vi "Facade.vi"(0 "Data In":T6={"t0"=timestamp(0 s since 1904-01-01), "dt"=0.0, "Y"=[]}, 2 "Display State In":T4, 3 "Container State":T5) -> (6 "Data Out":T6, 7 "Display State Out":T4, 8 "Action":T3)   [LabVIEW 2018, in "Waveform Control.xctl"]
uses:
  Waveform Control.xctl
  Controls/Data.ctl
  <vilib>/_xctls/Container State.ctl
  Controls/State.ctl
  <vilib>/_xctls/Action.ctl
  subvis/FP Controls.ctl
  subvis/Function Types.ctl
  Controls/Volatile State Ops.ctl
  <vilib>/_xctls/XControlSupport.lvlib
panel:
  in  "Controls":T1={"Type"=enum."Sine", "Periods"=0.0, "Points"=2, "Offset"=0.0, "Amplitdue"=0.0, "Starting Phase"=0.0, "func"=""} {"Points" min=1 step=1}
  out "Display":waveform(dbl)[](graph)
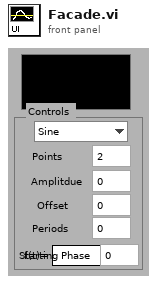
[diagram p1: front panel]
types:
  T1 = typedef "Waveform Control.xctl/FP Controls.ctl" = cluster{"Type":T2, "Periods":dbl, "Points":i32, "Offset":dbl, "Amplitdue":dbl, "Starting Phase":dbl, "func":string}
  T2 = typedef "Waveform Control.xctl/Function Types.ctl" = enum16{"Level", "Sine", "Triangle", "Ramp", "Saw Tooth", "Square", "Function"}
  T3 = typedef "XControlSupport.lvlib/Action.ctl" = cluster{"Data Changed?":bool, "State Changed?":bool, "Action Name":string}
  T4 = typedef "Waveform Control.xctl/State.ctl" = cluster{"Name":string}
  T5 = typedef "XControlSupport.lvlib/Container State.ctl" = cluster{"Indicator?":bool, "Run Mode?":bool, " Refnum":refnum<vi>}
  T6 = typedef "Waveform Control.xctl/Data.ctl" = waveform(dbl)
  T7 = typedef "Waveform Control.xctl/Volatile State Ops.ctl" = enum16{"Read", "Write", "Update State from Data"}
  T8 = typedef "Waveform Control.xctl/Waveform State.ctl" = cluster{"Show Axes":bool, "Show Y=0":bool, "Controls":T1, "Show Current Location":bool, "Current Location":i32, "dt":dbl, "t0":timestamp, "Amplitude Format String":string}
  T9 = typedef "LVRectTypeDef.ctl" = cluster{"Left":i16, "Top":i16, "Right":i16, "Bottom":i16}
  T10 = cluster{"Starting Phase":refnum<vi>, "Amplitdue":refnum<vi>, "Points":refnum<vi>, "Type":refnum<vi>, "Periods":refnum<vi>, "func":refnum<vi>, "Offset":refnum<vi>}
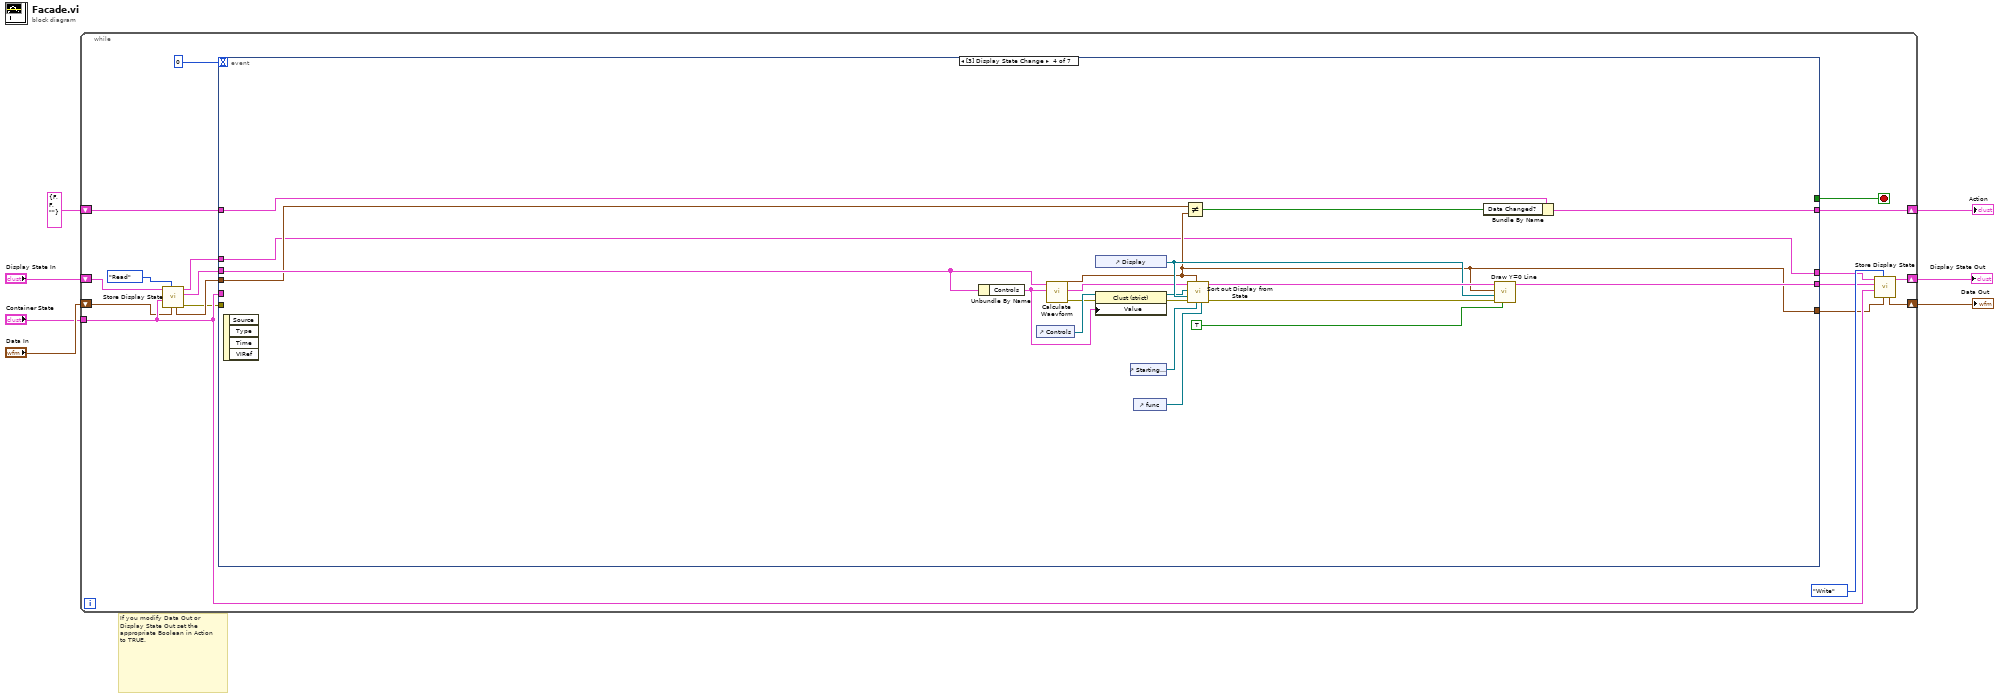
[diagram p0: block diagram]
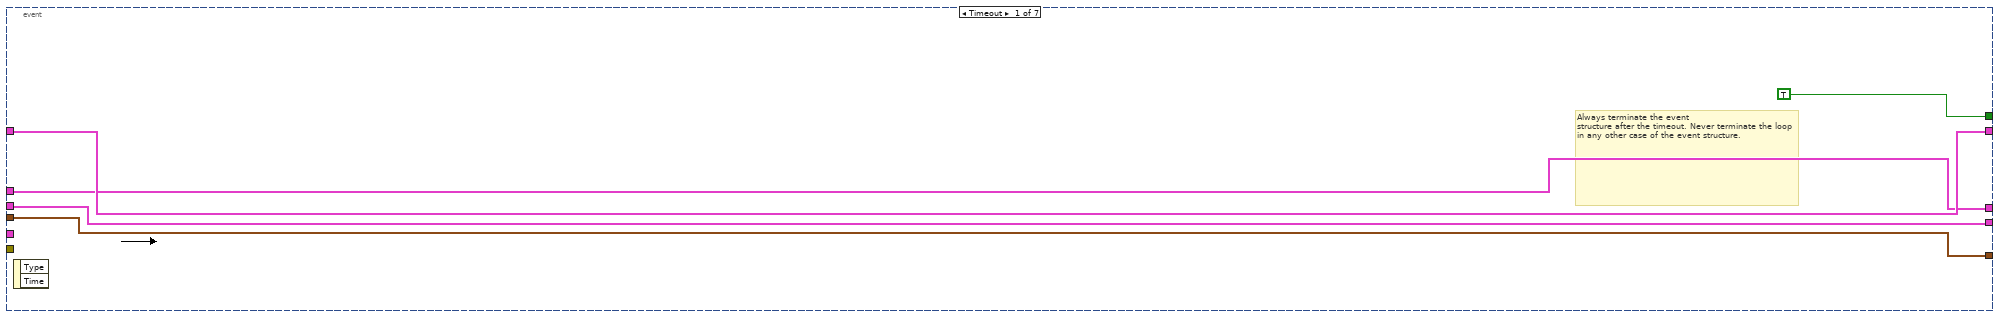
[diagram p2: hidden frame]
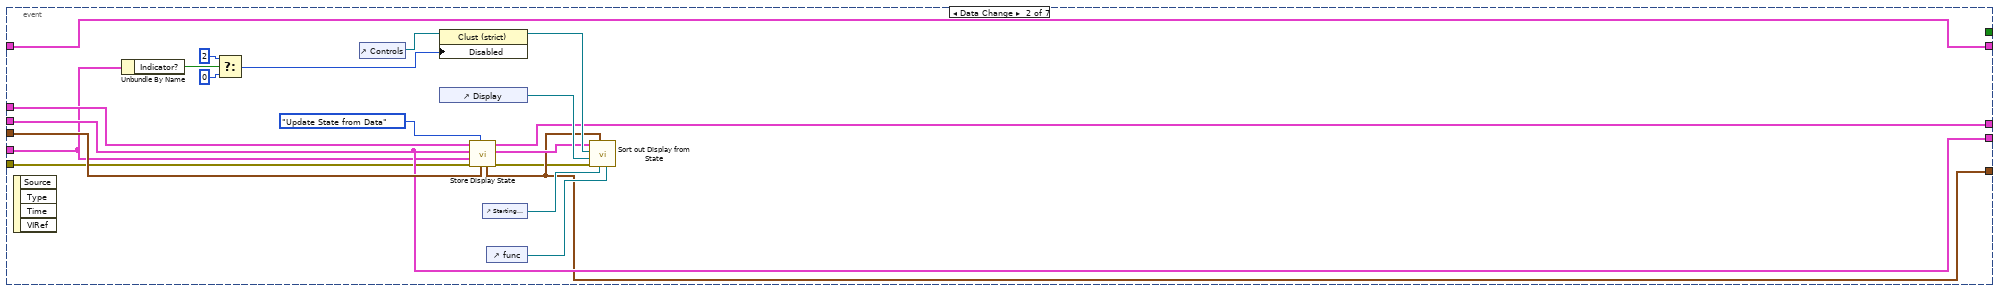
[diagram p3: hidden frame]
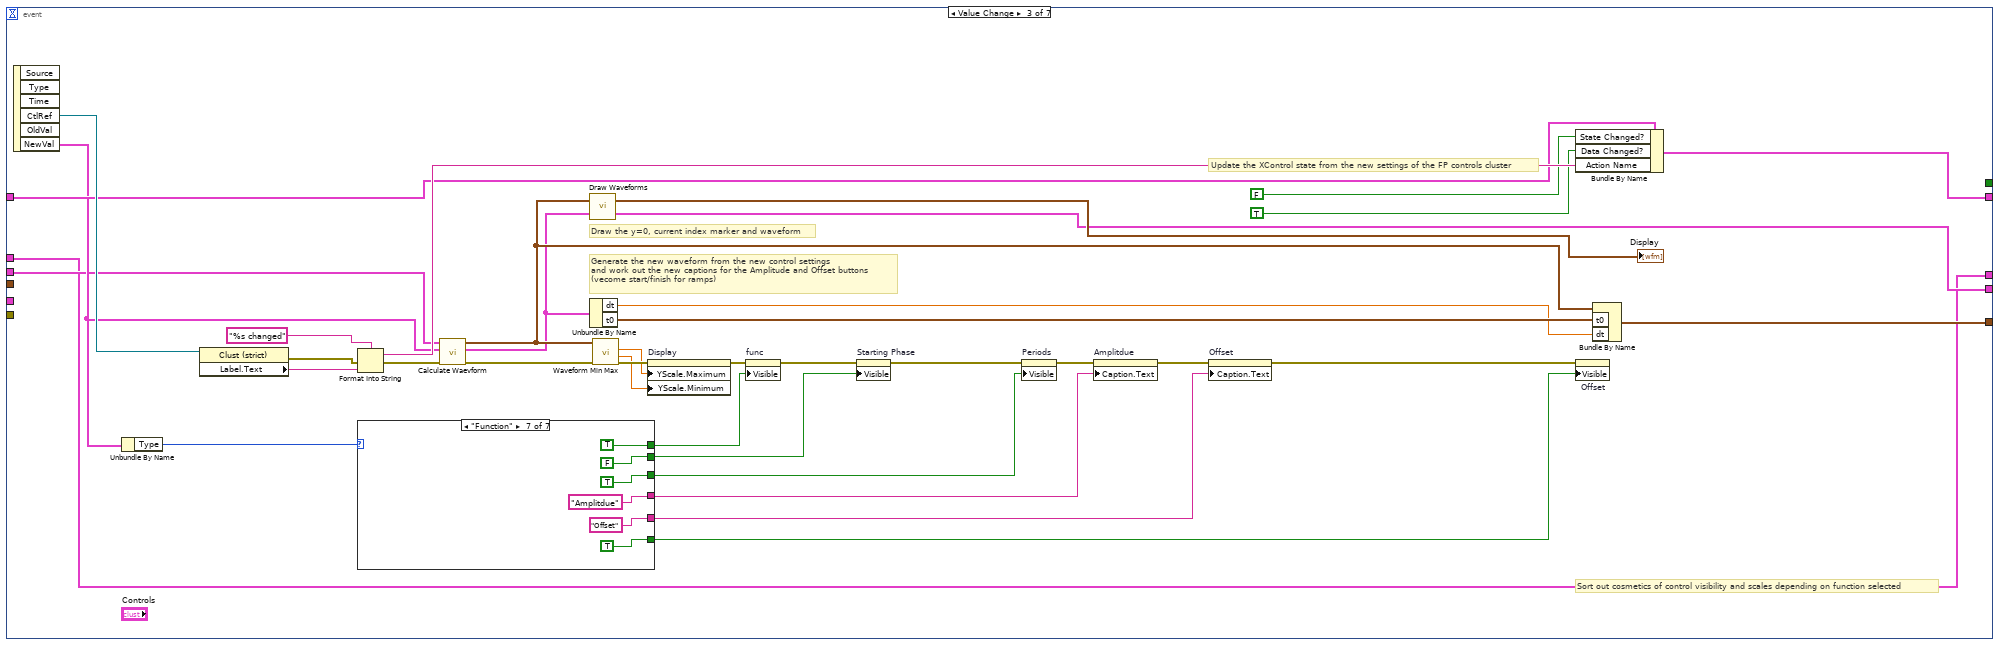
[diagram p4: hidden frame]
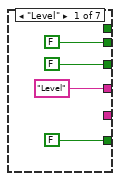
[diagram p5: hidden frame]
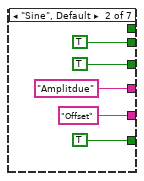
[diagram p6: hidden frame]
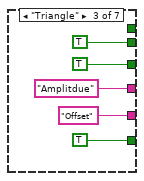
[diagram p7: hidden frame]
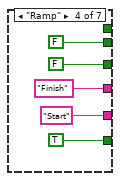
[diagram p8: hidden frame]
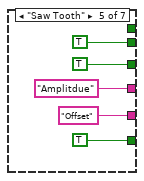
[diagram p9: hidden frame]
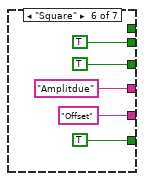
[diagram p10: hidden frame]
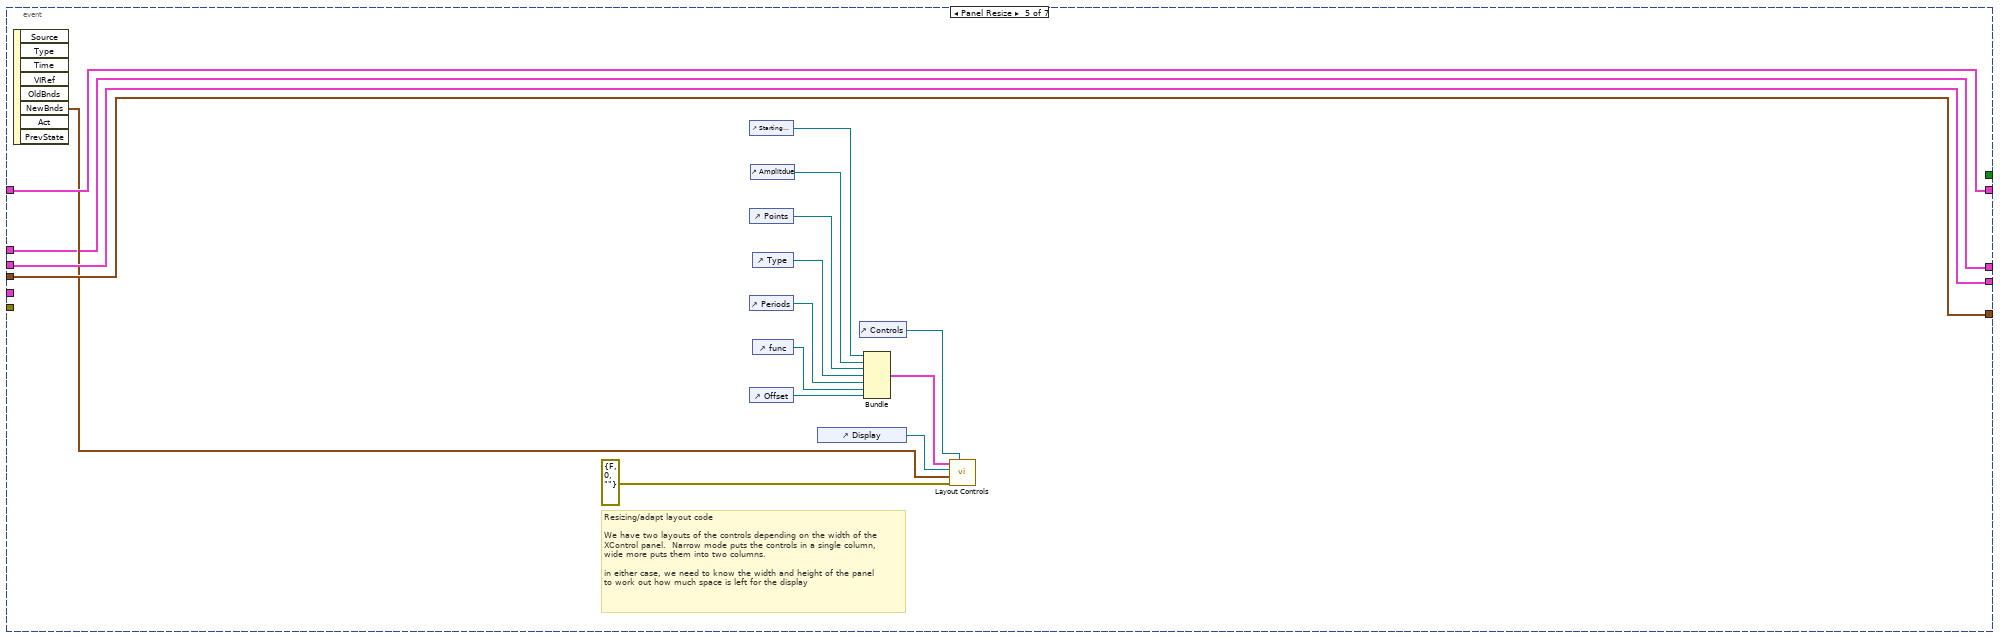
[diagram p11: hidden frame]
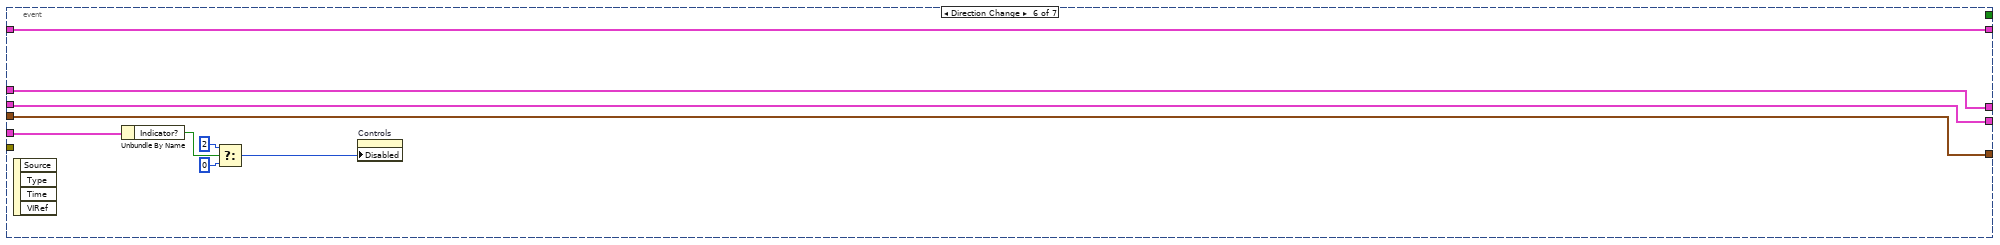
[diagram p12: hidden frame]
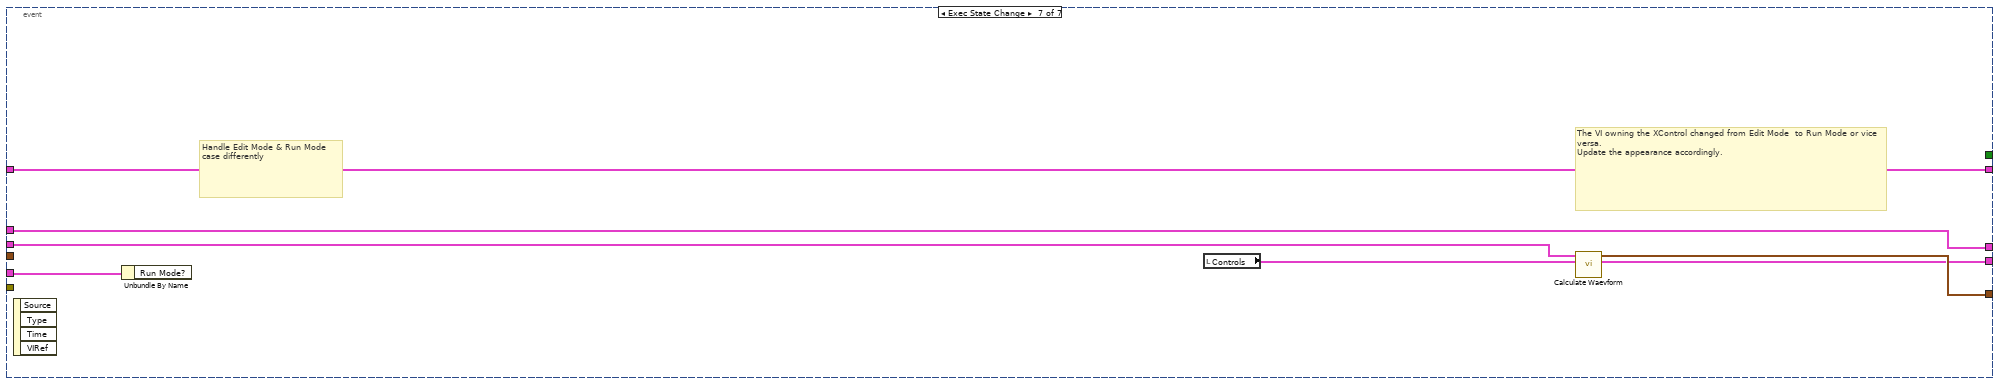
[diagram p13: hidden frame]
diagram:
  # "If you modify Data Out or\nDisplay State Out set the\nappropriate Boolean in Action\nto TRUE."
  n1 = while {
    shift-right: [w20] -> w4
    shift-left: "Display State In" -> [w25]
    tunnel: "Container State" -> [w15]
    shift-right: [w11] -> w7
    shift-left: "Data In" -> [w14]
    shift-right: [w21] -> w2
    shift-left: T3 {"Data Changed?"=FALSE, "State Changed?"=FALSE, "Action Name"=""} ("Action") -> [w22]
    stop <- w24 stop-if-true
    n2 = call "Store Display State.vi"("Data"=w14, "Operation In"=Volatile_State_Ops."Read", "Container State In"=w15, "State In"=w25) -> ("Error Out"=w8:errorcluster, "Waveform State Out"=w18:T8, "Display State Out"=w10:T4, "Data 2"=w13:T6)  [unwired: 2 in, 2 out]
    n3 = event shown="[3] Display State Change" {
      selector: _ -> [_ _ _ _ _ _ _]
      dyn-events: _ -> [_ _ _ _ _ _ _]
      timeout: 0 -> [_ _ _ _ _ _ _]
      tunnel: w18 -> [w28 w38 w54 w133 w157 w166 w169]
      tunnel: [w28 w38 w55 w134 w157 w166 w170] -> w17
      tunnel: [TRUE _ _ _ _ _ _] -> w24
      tunnel: w15 -> [_ w31 _ _ _ w167 w174]
      tunnel: w13 -> [w27 w40 _ w127 w158 w165 _]
      tunnel: [w27 w36 w62 w128 w158 w165 w171] -> w12
      tunnel: [w29 w32 w66 w141 w156 w164 w173] -> w21
      tunnel: w22 -> [w29 w32 w67 w142 w156 w164 w173]
      tunnel: w10 -> [w26 w41 w51 w125 w143 w159 w168]
      tunnel: [w26 w39 w51 w125 w143 w159 w168] -> w9
      tunnel: w8 -> [_ w33 _ _ _ _ _]
      event Timeout {
        # "Always terminate the event\nstructure after the timeout. Never terminate the loop in any other case of the event structure."
        n4 = event-data() -> ()  [unwired: 3 out]
      }
      event Data Change {
        n5 = event-data() -> ()  [unwired: 5 out]
        n6 = Unbundle By Name(w31) -> ("Indicator?"=w43:bool)
        n7 = Select(t=2, s=w43, f=0) -> (s? t:f=w46:i32)
        n8 = control-ref of="Controls"() -> (w50:refnum<vi>)
        n9 = property class="Clust (strict)"(reference=w50, "Disabled"=w46) -> (reference out=w42:refnum<vi>)  [unwired: 1 in, 1 out]
        n10 = control-ref of="Display"() -> (w47:refnum<vi>)
        n11 = call "Store Display State.vi"("Data"=w40, "Operation In"=Volatile_State_Ops."Update State from Data", "Error In (no Error) In"=w33, "Container State In"=w31, "Waveform State In"=w38, "State In"=w41) -> ("Error Out"=w34:errorcluster, "Waveform State Out"=w37:T8, "Display State Out"=w39:T4, "Data 2"=w36:T6)  [unwired: 2 out]
        n12 = control-ref of="Starting Phase"() -> (w48:refnum<vi>)
        n13 = control-ref of="func"() -> (w49:refnum<vi>)
        n14 = call "Sort out Display from State.vi"("func"=w49, "Starting Phase"=w48, "Data In"=w36, "error in (no error)"=w34, "Display"=w47, "Controls"=w42, "Display State In"=w37) -> ()  [unwired: 5 out]
      }
      event Value Change {
        # "Sort out cosmetics of control visibility and scales depending on function selected"
        # "Draw the y=0, current index marker and waveform"
        # "Generate the new waveform from the new control settings\nand work out the new captions for the Amplitude and Offset buttons\n(vecome start/finish for ramps)"
        # "Update the XControl state from the new settings of the FP controls cluster"
        n15 = event-data() -> ("CtlRef"=w87:refnum<vi>, "NewVal"=w60:T1)  [unwired: 5 out]
        n16 = Unbundle By Name(w60) -> ("Type"=w80:T2)
        n17 = property class="Clust (strict)"(reference=w87) -> (error out=w68:errorcluster, "Label.Text"=w85:string)  [unwired: 1 in, 1 out]
        n18 = Format Into String(format string="%s changed" ("Action Name"), error in=w68, w85) -> (resulting string=w84:string, error out=w58:errorcluster)  [unwired: 1 in]
        n19 = case shown="\"Function\"" w80 {
          tunnel: [_ _ _ _ _ _ TRUE] -> w79
          tunnel: [FALSE TRUE TRUE FALSE TRUE TRUE FALSE] -> w78
          tunnel: [FALSE TRUE TRUE FALSE TRUE TRUE TRUE] -> w77
          tunnel: ["Level" "Amplitdue" "Amplitdue" "Finish" "Amplitdue" "Amplitdue" "Amplitdue"] -> w76
          tunnel: [_ "Offset" "Offset" "Start" "Offset" "Offset" "Offset"] -> w75
          tunnel: [FALSE TRUE TRUE TRUE TRUE TRUE TRUE] -> w52
          frame "Level" {
          }
          frame "Sine", Default {
          }
          frame "Triangle" {
          }
          frame "Ramp" {
          }
          frame "Saw Tooth" {
          }
          frame "Square" {
          }
          frame "Function" {
          }
        }
        n20 = call "Calculate Waevform.vi"("error in (no error)"=w58, "Controls"=w60, "Display State In"=w54) -> ("error out"=w57:errorcluster, "Display State Out"=w56:T8, "signal out"=w59:waveform(dbl))  [unwired: 6 out]
        n21 = call "Draw Waveforms.vi"("Display State In"=w56, "Data In"=w59) -> ("Display State Out"=w55:T8, "Array"=→"Display":T6[])
        n22 = Unbundle By Name(w56) -> ("dt"=w64:dbl, "t0"=w65:timestamp)
        n23 = call <vilib>:"Waveform Min Max.vi"("error in (no error)"=w57, "waveform in"=w59) -> ("error out"=w83:errorcluster, "Y min"=w82:dbl, "Y max"=w81:dbl)  [unwired: 7 out]
        n24 = property on="Display" class="WFGraph (strict)"(error in=w83, "YScale.Maximum"=w81, "YScale.Minimum"=w82) -> (error out=w73:errorcluster)  [unwired: 1 in, 1 out]
        n25 = property on="func" class="Str"(error in=w73, "Visible"=w79) -> (error out=w72:errorcluster)  [unwired: 1 in, 1 out]
        n26 = property on="Starting Phase" class="DigNum (strict)"(error in=w72, "Visible"=w78) -> (error out=w71:errorcluster)  [unwired: 1 in, 1 out]
        n27 = property on="Periods" class="DigNum (strict)"(error in=w71, "Visible"=w77) -> (error out=w70:errorcluster)  [unwired: 1 in, 1 out]
        n28 = property on="Amplitdue" class="DigNum (strict)"(error in=w70, "Caption.Text"=w76) -> (error out=w69:errorcluster)  [unwired: 1 in, 1 out]
        n29 = property on="Offset" class="DigNum (strict)"(error in=w69, "Caption.Text"=w75) -> (error out=w53:errorcluster)  [unwired: 1 in, 1 out]
        n30 = Bundle By Name(cluster=w67, "State Changed?"=FALSE, "Data Changed?"=TRUE ("State Changed?"), "Action Name"=w84) -> (w66:T3)
        n31 = property on="Offset" class="DigNum (strict)"(error in=w53, "Visible"=w52) -> ()  [unwired: 1 in, 2 out]
        n32 = Bundle By Name(cluster=w59, "t0"=w65, "dt"=w64) -> (w62:waveform(dbl))
      }
      event Display State Change {
        n33 = event-data() -> ()  [unwired: 5 out]
        n34 = Unbundle By Name(w133) -> ("Controls"=w123:T1)
        n35 = control-ref of="Controls"() -> (w132:refnum<vi>)
        n36 = call "Calculate Waevform.vi"("Controls"=w123, "Display State In"=w133) -> ("error out"=w124:errorcluster, "Display State Out"=w131:T8, "signal out"=w128:waveform(dbl))  [unwired: 1 in, 6 out]
        n37 = control-ref of="Display"() -> (w136:refnum<vi>)
        n38 = property class="Clust (strict)"(reference=w132, error in=w124, "Value"=w123) -> (reference out=w129:refnum<vi>, error out=w130:errorcluster)
        n39 = control-ref of="Starting Phase"() -> (w139:refnum<vi>)
        n40 = control-ref of="func"() -> (w140:refnum<vi>)
        n41 = Not Equal?(x=w127, y=w128) -> (x != y?=w126:bool)
        n42 = call "Sort out Display from State.vi"("func"=w140, "Starting Phase"=w139, "Data In"=w128, "error in (no error)"=w130, "Display"=w136, "Controls"=w129, "Display State In"=w131) -> ("errorout"=w138:errorcluster, "Display State In 2"=w137:T8)  [unwired: 3 out]
        n43 = Bundle By Name(cluster=w142, "Data Changed?"=w126) -> (w141:T3)
        n44 = call "Draw Y=0 Line.vi"("Needs update"=TRUE, "error in (no error)"=w138, "PreviewGraph Ref"=w136, "Data In"=w128, "Display State In"=w137) -> ("Display State Out"=w134:T8)  [unwired: 2 in, 4 out]
      }
      event Panel Resize {
        # "Resizing/adapt layout code\n\nWe have two layouts of the controls depending on the width of the\nXControl panel.  Narrow mode puts the controls in a single column,\nwide more puts them into two columns.\n\nin either case, we need to know the width and height of the panel\nto work out how much space is left for the display"
        n45 = event-data() -> ("NewBnds"=w146:T9)  [unwired: 8 out]
        n46 = control-ref of="Starting Phase"() -> (w155:refnum<vi>)
        n47 = control-ref of="Points"() -> (w153:refnum<vi>)
        n48 = control-ref of="Periods"() -> (w151:refnum<vi>)
        n49 = control-ref of="Offset"() -> (w149:refnum<vi>)
        n50 = control-ref of="Amplitdue"() -> (w154:refnum<vi>)
        n51 = control-ref of="Type"() -> (w152:refnum<vi>)
        n52 = control-ref of="func"() -> (w150:refnum<vi>)
        n53 = control-ref of="Display"() -> (w147:refnum<vi>)
        n54 = control-ref of="Controls"() -> (w144:refnum<vi>)
        n55 = Bundle("Starting Phase"=w155, "Amplitdue"=w154, "Points"=w153, "Type"=w152, "Periods"=w151, "func"=w150, "Offset"=w149) -> (w145:T10)  [unwired: 1 out]
        n56 = call "Layout Controls.vi"("Control Cliuster"=w144, "error out"=errorcluster {"status"=FALSE, "code"=0, "source"=""}, "NewBnds"=w146, "Waveform Ref"=w147, "Controls Refs"=w145) -> ()  [unwired: 4 in, 3 out]
      }
      event Direction Change {
        n57 = event-data() -> ()  [unwired: 5 out]
        n58 = Unbundle By Name(w167) -> ("Indicator?"=w163:bool)
        n59 = Select(t=2, s=w163, f=0) -> (s? t:f=w160:i32)
        n60 = property on="Controls" class="Clust (strict)"("Disabled"=w160) -> ()  [unwired: 2 in, 2 out]
      }
      event Exec State Change {
        # "The VI owning the XControl changed from Edit Mode  to Run Mode or vice versa.\nUpdate the appearance accordingly."
        # "Handle Edit Mode & Run Mode\ncase differently"
        n61 = event-data() -> ()  [unwired: 5 out]
        n62 = Unbundle By Name(w174) -> ()  [unwired: 1 out]
        n63 = local read "Controls"() -> (w172:T1)
        n64 = call "Calculate Waevform.vi"("Controls"=w172, "Display State In"=w169) -> ("Display State Out"=w170:T8, "signal out"=w171:waveform(dbl))  [unwired: 1 in, 7 out]
      }
    }
    n65 = call "Store Display State.vi"("Data"=w12, "Operation In"=Volatile_State_Ops."Write", "Container State In"=w15, "Waveform State In"=w17, "State In"=w9) -> ("Display State Out"=w20:T4, "Data 2"=w11:T6)  [unwired: 1 in, 4 out]
  }
  "Display State Out" <- w4
  "Data Out" <- w7
  "Action" <- w2
